vi "GV subtrigger.vi"() -> ()   [LabVIEW 2017]
panel:
  out "Subtrigger":bool
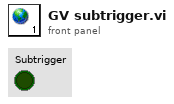
[diagram p1: front panel]
diagram:
